vi "Send to Behavior Classifier (SubVI).vi"(0 "DLL Input Param":T1={"DateTimeStamp"="DateTimeStamp", "Genotype 1"="genotype1", "Genotype 2"="genotype2", "Rig Name"="stimulationMode", "STIM Mode"="t21", "Light Intensity (%)"=100, "Pixel Resolution (um/pixel)"=100.0, "Gamma"=0.2, "Yoked File Name"="none", "Yoked File Enable"=FALSE, "Output Folder Name"=path "", "Frame Number"=0, "Time Stamp (us)"=0, "Exp STOP"=0, "Contour"=[], "SPINE"=[], "Larvae ID"=[], "Larvae Valid?"=[], "Image Height"=0, "Image Width"=0, "Pixel Intensity Low"=0, "Pixel Intensity High"=0, "Box Side Low"=0, "Box Side High"=0, "Box W+L Low"=0, "Box W+L High"=0, "Area Low"=0, "Area High"=0, "N SPINE"=0, "BG SUB TH"=0, "Min Contour Points"=0, "STIM Array"=[], "Stimulus Label Array"=[], "Flip Laravae ID"=[], "IR Intensity"=0}) -> (14 "dmdData":i32[](array[numeric]), 15 "voteRESET":u32[][](array[numeric]), 16 "irData":i32[](array[numeric]))   [LabVIEW 2020]
uses:
  Controls (HOST)/File Name Prefix.ctl
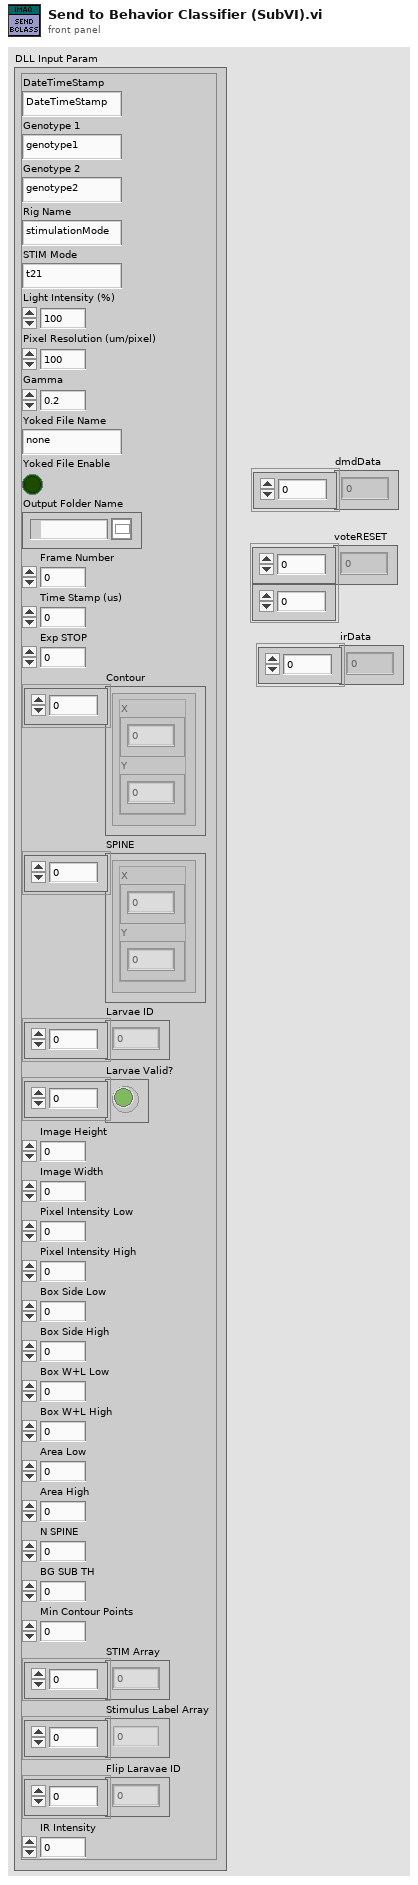
[diagram p1: front panel]
types:
  T1 = typedef "File Name Prefix.ctl" = cluster{"DateTimeStamp":string, "Genotype 1":string, "Genotype 2":string, "Rig Name":string, "STIM Mode":string, "Light Intensity (%)":i32, "Pixel Resolution (um/pixel)":dbl, "Gamma":dbl, "Yoked File Name":string, "Yoked File Enable":bool, "Output Folder Name":path, "Frame Number":u64, "Time Stamp (us)":u64, "Exp STOP":i32, "Contour":cluster{"X":i32[], "Y":i32[]}[], "SPINE":cluster{"X":dbl[], "Y":dbl[]}[], "Larvae ID":u32[], "Larvae Valid?":bool[], "Image Height":i32, "Image Width":i32, "Pixel Intensity Low":i32, "Pixel Intensity High":i32, "Box Side Low":i32, "Box Side High":i32, "Box W+L Low":i32, "Box W+L High":i32, "Area Low":i32, "Area High":i32, "N SPINE":i32, "BG SUB TH":i32, "Min Contour Points":i32, "STIM Array":dbl[], "Stimulus Label Array":u8[], "Flip Laravae ID":i32[], "IR Intensity":i32}
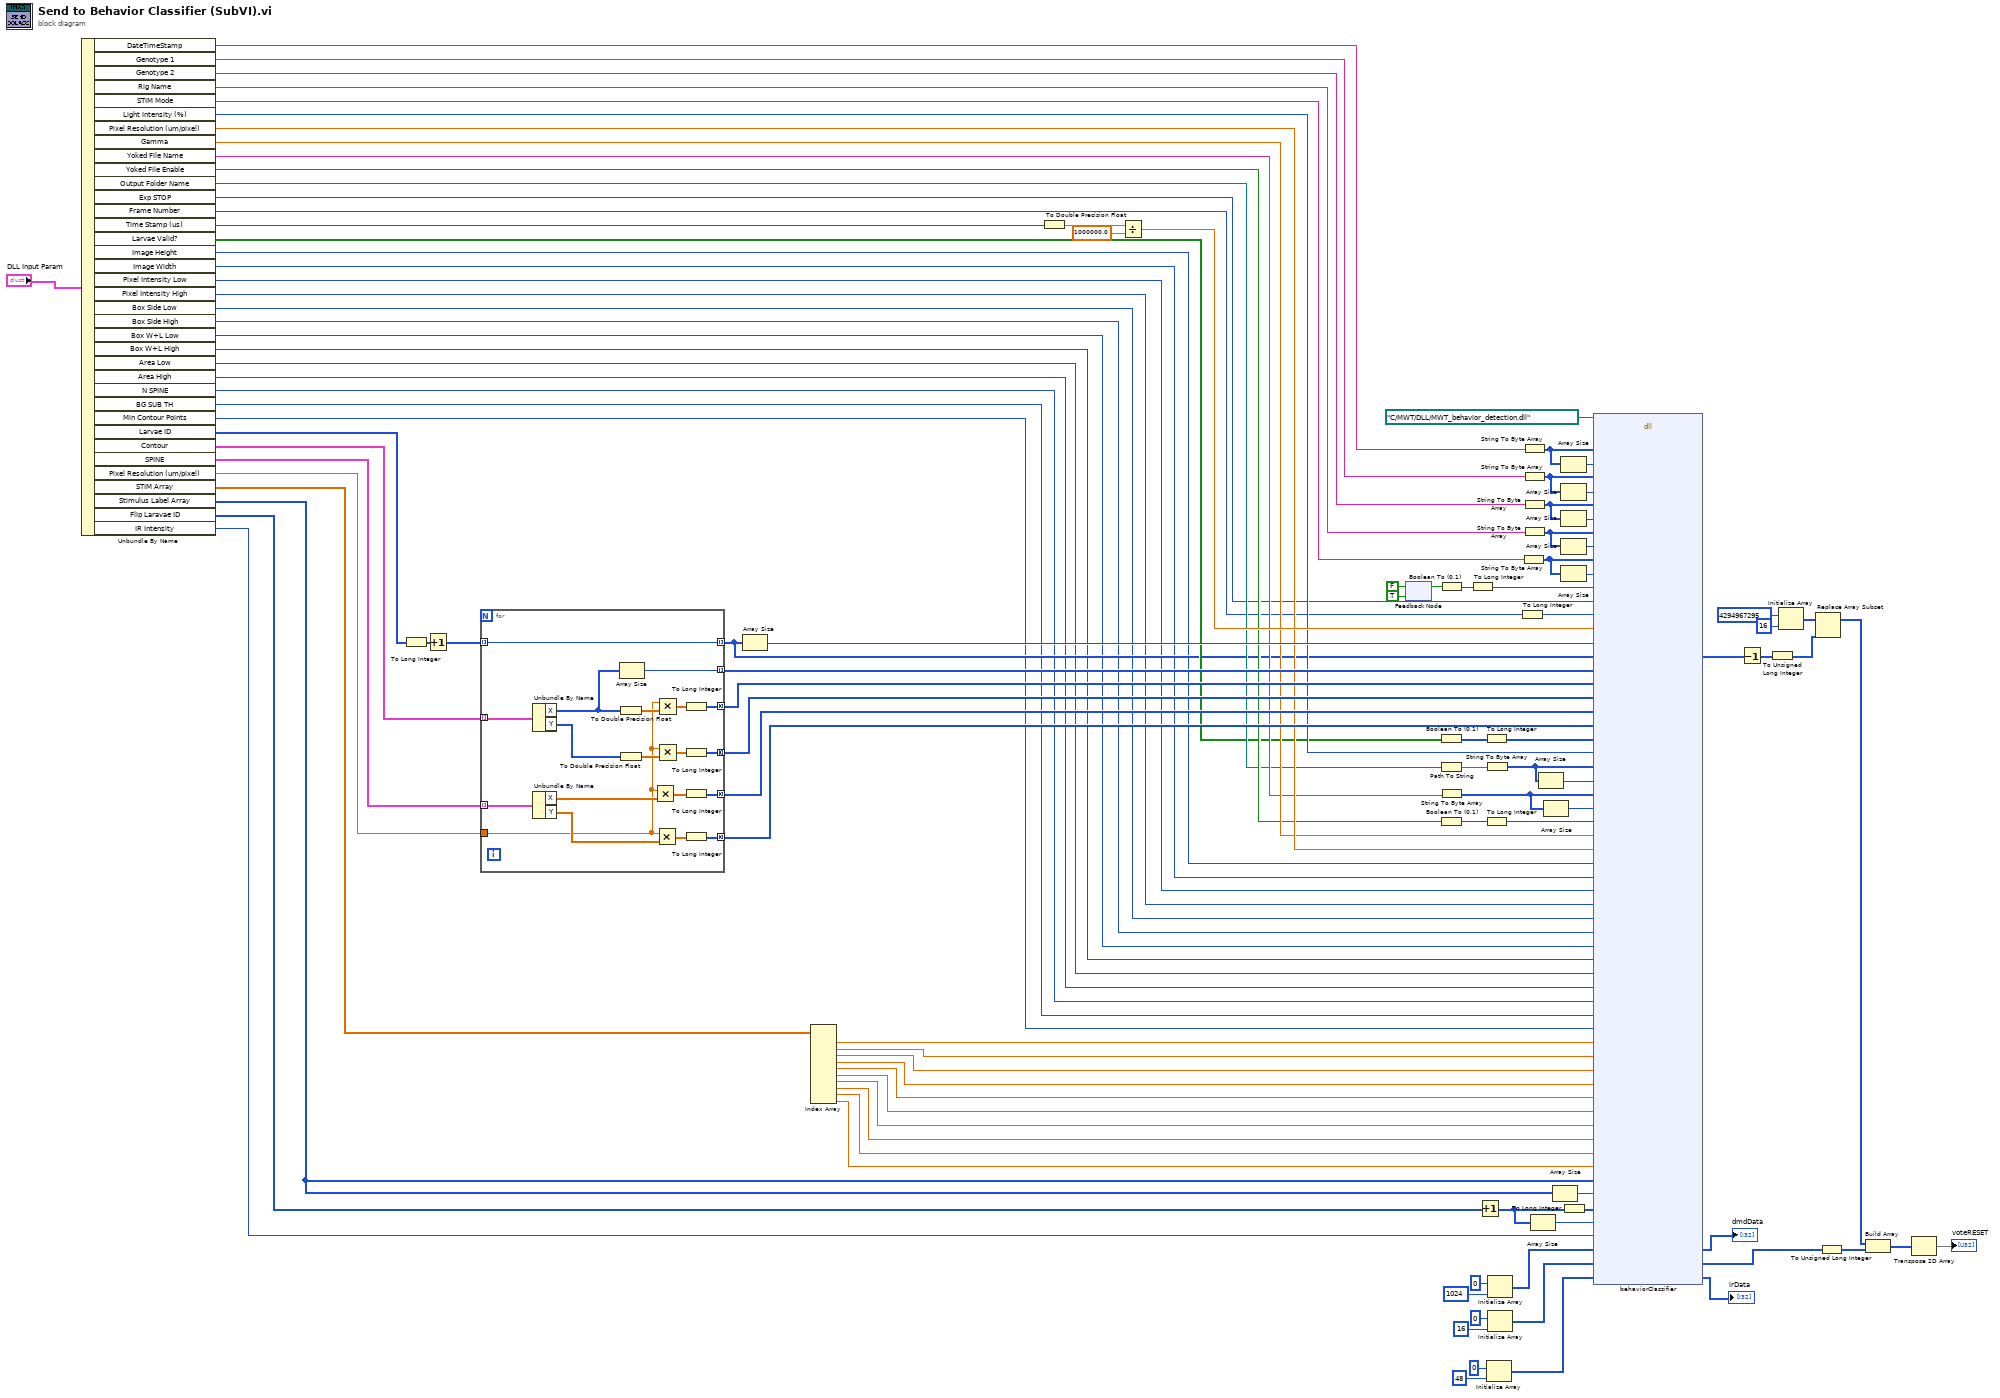
[diagram p0: block diagram]
diagram:
  n1 = Unbundle By Name("DLL Input Param") -> ("DateTimeStamp"=w82:string, "Genotype 1"=w81:string, "Genotype 2"=w80:string, "Rig Name"=w79:string, "STIM Mode"=w78:string, "Light Intensity (%)"=w77:i32, "Pixel Resolution (um/pixel)"=w64:dbl, "Gamma"=w63:dbl, "Yoked File Name"=w62:string, "Yoked File Enable"=w61:bool, "Output Folder Name"=w60:path, "Exp STOP"=w59:i32, "Frame Number"=w8:u64, "Time Stamp (us)"=w7:u64, "Larvae Valid?"=w58:bool[], "Image Height"=w52:i32, "Image Width"=w51:i32, "Pixel Intensity Low"=w50:i32, "Pixel Intensity High"=w49:i32, "Box Side Low"=w48:i32, "Box Side High"=w47:i32, "Box W+L Low"=w46:i32, "Box W+L High"=w45:i32, "Area Low"=w44:i32, "Area High"=w43:i32, "N SPINE"=w42:i32, "BG SUB TH"=w41:i32, "Min Contour Points"=w40:i32, "Larvae ID"=w55:u32[], "Contour"=w57:cluster{"X":i32[], "Y":i32[]}[], "SPINE"=w56:cluster{"X":dbl[], "Y":dbl[]}[], "Pixel Resolution (um/pixel)"=w54:dbl, "STIM Array"=w39:dbl[], "Stimulus Label Array"=w28:u8[], "Flip Laravae ID"=w12:i32[], "IR Intensity"=w1:i32)
  n2 = To Long Integer(number=w55) -> (32bit integer=w107:i32[])
  n3 = Increment(x=w107) -> (x+1=w99:i32[])
  n4 = for {
    tunnel: w56 -> [w130] mode=indexing
    tunnel: w57 -> [w128] mode=indexing
    tunnel: [w118] -> w108 mode=concatenating
    tunnel: [w117] -> w109 mode=concatenating
    tunnel: [w116] -> w110 mode=concatenating
    tunnel: [w115] -> w111 mode=concatenating
    tunnel: [w119] -> w106 mode=indexing
    tunnel: w99 -> [w114] mode=indexing
    tunnel: [w114] -> w53 mode=indexing
    tunnel: w54 -> [w112]
    n5 = Unbundle By Name(w128) -> ("X"=w120:i32[], "Y"=w127:i32[])
    n6 = Unbundle By Name(w130) -> ("X"=w129:dbl[], "Y"=w113:dbl[])
    n7 = To Double Precision Float(number=w120) -> (double precision float=w126:dbl[])
    n8 = To Double Precision Float(number=w127) -> (double precision float=w125:dbl[])
    n9 = Array Size(array=w120) -> (size(s)=w119:i32)
    n10 = Multiply(x=w112, y=w129) -> (x*y=w124:dbl[])
    n11 = Multiply(x=w112, y=w113) -> (x*y=w123:dbl[])
    n12 = Multiply(x=w112, y=w126) -> (x*y=w122:dbl[])
    n13 = Multiply(x=w112, y=w125) -> (x*y=w121:dbl[])
    n14 = To Long Integer(number=w122) -> (32bit integer=w116:i32[])
    n15 = To Long Integer(number=w121) -> (32bit integer=w115:i32[])
    n16 = To Long Integer(number=w124) -> (32bit integer=w118:i32[])
    n17 = To Long Integer(number=w123) -> (32bit integer=w117:i32[])
  }
  n18 = Array Size(array=w53) -> (size(s)=w105:i32)
  n19 = Index Array(array=w39) -> (element #1=w38:dbl, element #2=w37:dbl, element #3=w36:dbl, element #4=w35:dbl, element #5=w34:dbl, element #6=w33:dbl, element #7=w32:dbl, element #8=w31:dbl, element #9=w30:dbl, element #10=w29:dbl)  [unwired: 10 in]
  n20 = To Double Precision Float(number=w7) -> (double precision float=w103:dbl)
  n21 = Divide(x=w103, y=1000000.0) -> (x/y=w101:dbl)
  n22 = feedback #1(TRUE) -> (w86:bool)
  n23 = feedback-in #1(FALSE) -> ()
  n24 = Boolean To (0,1)(Boolean=w58) -> (0, 1=w76:i16[])
  n25 = Path To String(path=w60) -> (string=w74:string)
  n26 = Boolean To (0,1)(Boolean=w61) -> (0, 1=w73:i16)
  n27 = Boolean To (0,1)(Boolean=w86) -> (0, 1=w85:i16)
  n28 = String To Byte Array(string=w62) -> (unsigned byte array=w68:u8[])
  n29 = To Long Integer(number=w85) -> (32bit integer=w84:i32)
  n30 = Increment(x=w12) -> (x+1=w11:i32[])
  n31 = To Long Integer(number=w76) -> (32bit integer=w75:i32[])
  n32 = To Long Integer(number=w73) -> (32bit integer=w72:i32)
  n33 = String To Byte Array(string=w74) -> (unsigned byte array=w71:u8[])
  n34 = Initialize Array(0 ("element"), 48 ("dimension size")) -> (w3:i32[])
  n35 = Initialize Array(0 ("element"), 1024 ("dimension size")) -> (w26:i32[])
  n36 = Initialize Array(0 ("element"), 16 ("dimension size")) -> (w23:i32[])
  n37 = To Long Integer(number=w8) -> (32bit integer=w100:i32)
  n38 = String To Byte Array(string=w78) -> (unsigned byte array=w89:u8[])
  n39 = String To Byte Array(string=w82) -> (unsigned byte array=w97:u8[])
  n40 = String To Byte Array(string=w81) -> (unsigned byte array=w95:u8[])
  n41 = String To Byte Array(string=w80) -> (unsigned byte array=w93:u8[])
  n42 = String To Byte Array(string=w79) -> (unsigned byte array=w91:u8[])
  n43 = Array Size(array=w11) -> (size(s)=w13:i32)
  n44 = Array Size(array=w71) -> (size(s)=w70:i32)
  n45 = Array Size(array=w68) -> (size(s)=w69:i32)
  n46 = Array Size(array=w28) -> (size(s)=w27:i32)
  n47 = Array Size(array=w97) -> (size(s)=w98:i32)
  n48 = Array Size(array=w95) -> (size(s)=w96:i32)
  n49 = Array Size(array=w93) -> (size(s)=w94:i32)
  n50 = Array Size(array=w91) -> (size(s)=w92:i32)
  n51 = Array Size(array=w89) -> (size(s)=w90:i32)
  n52 = To Long Integer(number=w11) -> (32bit integer=w14:i32[])
  n53 = dll-call lib="C:/MWT/DLL/MWT_behavior_detection.dll" fn="behaviorClassifier"(path in=path "C:/MWT/DLL/MWT_behavior_detection.dll", "dateTime"=w97, "dateTimeLen"=w98, "Genotype1"=w95, "genotype1Len"=w96, "Genotype2"=w93, "genotype2Len"=w94, "StimulationMode"=w91, "stimModeLen"=w92, "RigName"=w89, "rigNameLen"=w90, "experimentStart"=w84, "experimentStop"=w59, "frameNum"=w100, "timeStamp"=w101, "numLarvae"=w105, "larvaeIDs"=w53, "nContour"=w106, "xContour"=w110, "yContour"=w111, "xSpine"=w108, "ySpine"=w109, "LarvaeValid"=w75, "Intensity"=w77, "FolderName"=w71, "FolderNameLen"=w70, "YokedFileName"=w68, "YokedFileNameLen"=w69, "YokedFileEnable"=w72, "Gamma"=w63, "pixelResolution"=w64, "ImageHeight"=w52, "ImageWidth"=w51, "PixelIntensityLow"=w50, "PixelIntensityHigh"=w49, "BoxSideLow"=w48, "BoxSideHigh"=w47, "BowW+LLow"=w46, "BoxW+LHigh"=w45, "AreaLow"=w44, "AreaHigh"=w43, "NSpine"=w42, "BGSubTH"=w41, "MinContourPoints"=w40, "STIM1"=w38, "STIM2"=w37, "STIM3"=w36, "STIM4"=w35, "STIM5"=w34, "STIM6"=w33, "STIM7"=w32, "STIM8"=w31, "STIM9"=w30, "STIM10"=w29, "StimLabels"=w28, "StimLabelsLen"=w27, "flipLarvaeID"=w14, "flipFlagLen"=w13, "IRIntensity"=w1, "dmdData"=w26, "voteReset"=w23, "irData"=w3) -> ("larvaeIDs"=w17:i32[], "dmdData"=→"dmdData":i32[], "voteReset"=w25:i32[], "irData"=→"irData":i32[])  [unwired: 60 in, 2 out]
  n54 = Decrement(x=w17) -> (x-1=w15:i32[])
  n55 = To Unsigned Long Integer(number=w15) -> (unsigned 32bit integer=w16:u32[])
  n56 = Initialize Array(u32 4294967295 ("element"), 16 ("dimension size")) -> (w18:u32[])
  n57 = Replace Array Subset(array=w18, new element=w16) -> (w10:u32[])  [unwired: 1 in]
  n58 = To Unsigned Long Integer(number=w25) -> (unsigned 32bit integer=w9:u32[])
  n59 = Build Array(w10, w9) -> (w19:u32[][])
  n60 = Transpose 2D Array(2D array=w19) -> (transposed array=→"voteRESET":u32[][])
